vi "Configure DC Volts4.vi"(8 "error in (no error)":errorcluster, 10 "measurementservice_DMMConfigRequest_Data":T1) -> (0 "error out":errorcluster, 2 "measurementservice_DMMConfigRequest_Data Out":T1)   [LabVIEW 2019, in "HVC4.lvlib" / "HVC4.lvclass"]
uses:
  HVC4 Class/HVC4.lvclass
  <instrlib>/niDMM/nidmm.llb/niDMM Configure Measurement Digits.vi
  <instrlib>/niDMM/nidmm.llb/niDMM Control Actions.ctl
  HVC4 Class/RPC Messages/measurementservice_DMMConfigRequest/measurementservice_DMMConfigRequest_Data.ctl
panel:
  in  "DMM Function Array":i32[](array[numeric])=[1, 2, 3, 4, 5, 101, 1002, 104, 105, 1001, 1005, 1006, 108]
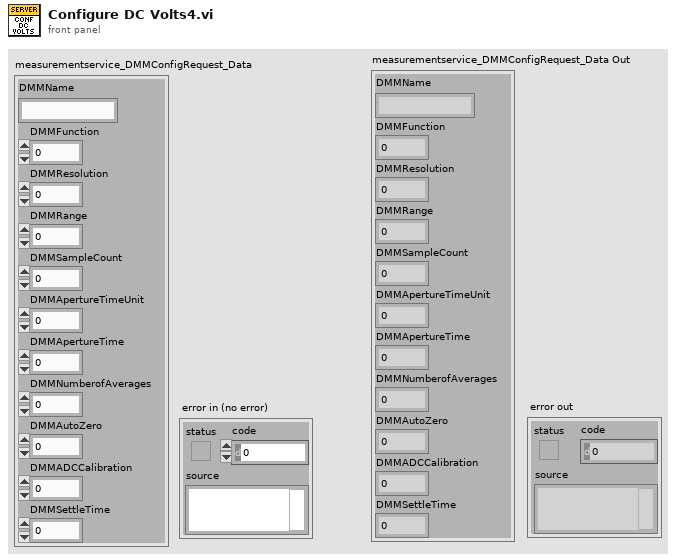
[diagram p1: front panel]
types:
  T1 = typedef "HVC4.lvlib/HVC4.lvclass/measurementservice_DMMConfigRequest_Data.ctl" = cluster{"DMMName":string, "DMMFunction":i32, "DMMResolution":sgl, "DMMRange":sgl, "DMMSampleCount":i32, "DMMApertureTimeUnit":i32, "DMMApertureTime":sgl, "DMMNumberofAverages":i32, "DMMAutoZero":i32, "DMMADCCalibration":i32, "DMMSettleTime":sgl}
  T2 = typedef "niDMM Control Actions.ctl" = i32
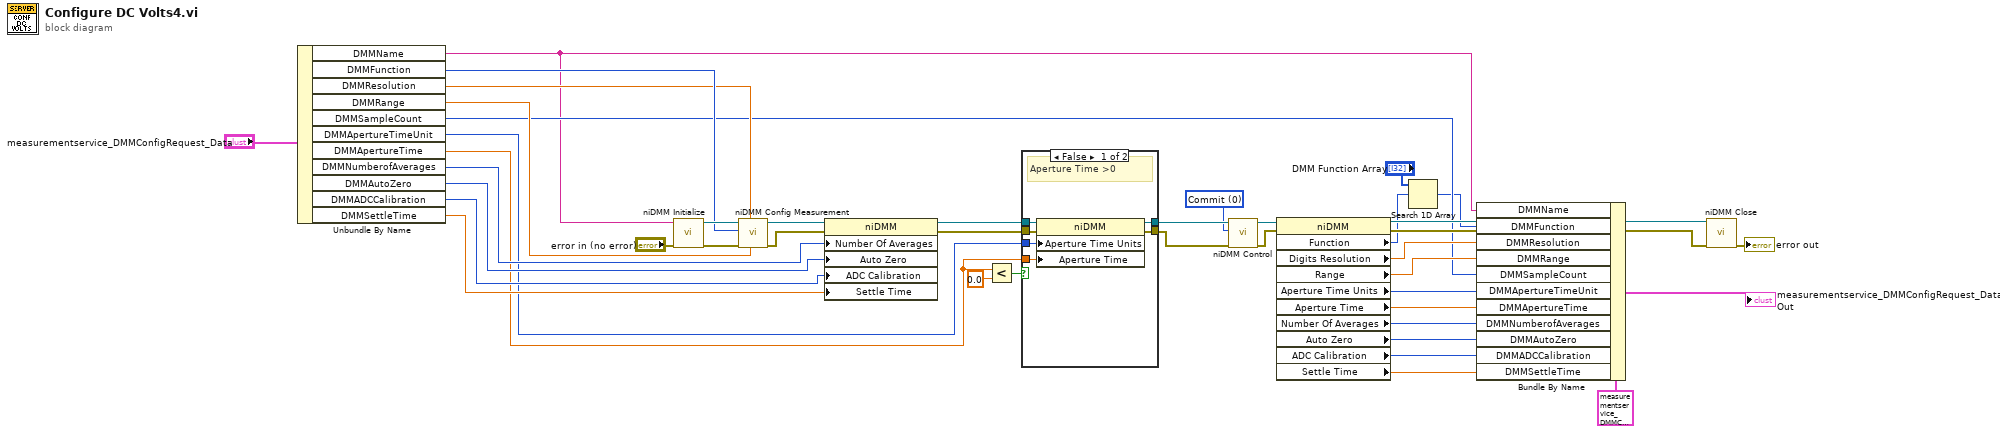
[diagram p0: block diagram]
diagram:
  w22 = T2 0 items=["Commit"] ("Control Action")
  n1 = Unbundle By Name("measurementservice_DMMConfigRequest_Data") -> ("DMMName"=w2:string, "DMMFunction"=w39:i32, "DMMResolution"=w38:sgl, "DMMRange"=w37:sgl, "DMMSampleCount"=w9:i32, "DMMApertureTimeUnit"=w26:i32, "DMMApertureTime"=w25:sgl, "DMMNumberofAverages"=w34:i32, "DMMAutoZero"=w33:i32, "DMMADCCalibration"=w32:i32, "DMMSettleTime"=w31:sgl)
  n2 = call <instrlib>:"niDMM Initialize.vi"("error in (no error)"="error in (no error)", "Instrument Descriptor"=w2) -> ("error out"=w40:errorcluster, "instrument handle out"=w41:refnum<k15>)  [unwired: 8 in]
  n3 = call-poly <instrlib>:"niDMM Config Measurement.vi"("Range"=w37, "Resolution in Digits"=w38, "error in (no error)"=w40, "Function"=w39, "instrument handle"=w41) -> ("error out"=w35:errorcluster, "instrument handle out"=w36:refnum<k15>)  [unwired: 5 in]
  n4 = property class="niDMM"(reference=w36, error in=w35, "Number Of Averages"=w34, "Auto Zero"=w33, "ADC Calibration"=w32, "Settle Time"=w31) -> (reference out=w30:refnum<k15>, error out=w29:errorcluster)
  n5 = Less?(x=w25, y=0.0 ("Configuration:Advanced:Aperture Time")) -> (x < y?=w27:bool)
  n6 = case shown="False" w27 {
    tunnel: w30 -> [w48 w50]
    tunnel: w29 -> [w47 w49]
    tunnel: [w46 w50] -> w24
    tunnel: [w45 w49] -> w23
    tunnel: w26 -> [w44 _]
    tunnel: w25 -> [w43 _]
    frame False {
      # "Aperture Time >0"
      n7 = property class="niDMM"(reference=w48, error in=w47, "Aperture Time Units"=w44, "Aperture Time"=w43) -> (reference out=w46:refnum<k15>, error out=w45:errorcluster)
    }
    frame True {
      # "Aperture Time <0"
    }
  }
  n8 = call <instrlib>:"niDMM Control.vi"("error in (no error)"=w23, "Control Action"=w22, "instrument handle"=w24) -> ("error out"=w20:errorcluster, "instrument handle out"=w21:refnum<k15>)  [unwired: 7 in]
  n9 = property class="niDMM"(reference=w21, error in=w20) -> (reference out=w19:refnum<k15>, error out=w18:errorcluster, "Function"=w7:i32, "Digits Resolution"=w10:dbl, "Range"=w11:dbl, "Aperture Time Units"=w12:i32, "Aperture Time"=w13:dbl, "Number Of Averages"=w14:i32, "Auto Zero"=w15:i32, "ADC Calibration"=w16:i32, "Settle Time"=w17:dbl)
  n10 = Search 1D Array(1D array="DMM Function Array", element=w7) -> (index of element=w6:i32)  [unwired: 1 in]
  n11 = Bundle By Name(cluster=T1 {"DMMName"="", "DMMFunction"=0, "DMMResolution"=0.0, "DMMRange"=0.0, "DMMSampleCount"=0, "DMMApertureTimeUnit"=0, "DMMApertureTime"=0.0, "DMMNumberofAverages"=0, "DMMAutoZero"=0, "DMMADCCalibration"=0, "DMMSettleTime"=0.0} ("measurementservice_DMMConfigRequest_Data Out"), "DMMName"=w2, "DMMFunction"=w6, "DMMResolution"=w10, "DMMRange"=w11, "DMMSampleCount"=w9, "DMMApertureTimeUnit"=w12, "DMMApertureTime"=w13, "DMMNumberofAverages"=w14, "DMMAutoZero"=w15, "DMMADCCalibration"=w16, "DMMSettleTime"=w17) -> (→"measurementservice_DMMConfigRequest_Data Out":T1)
  n12 = call <instrlib>:"niDMM Close.vi"("error in (no error)"=w18, "instrument handle"=w19) -> ("error out"=→"error out":errorcluster)  [unwired: 9 in]
